vi "Interpolation Example.vi"() -> ()   [LabVIEW 2018]
uses:
  <vilib>/Analysis/1siggen.llb/Ramp Pattern by Samples.vi
  <vilib>/gmath/NI_Gmath.lvlib
  <vilib>/Analysis/NI_AALBase.lvlib
panel:
  out "Raw outputs":cluster{"X":dbl[], "Y":dbl[]}
  in  "samples":i32=256
  in  "method":i32(ring)=1 items=["nearest", "linear", "spline", "cubic Hermite", "Lagrange"]
  in  "Y":dbl[](array[slide]) scale=0.0..1.0
  in  "On/Off":bool
  out "Output Values":cluster{"xi used":dbl[], "yi":dbl[]}(graph)
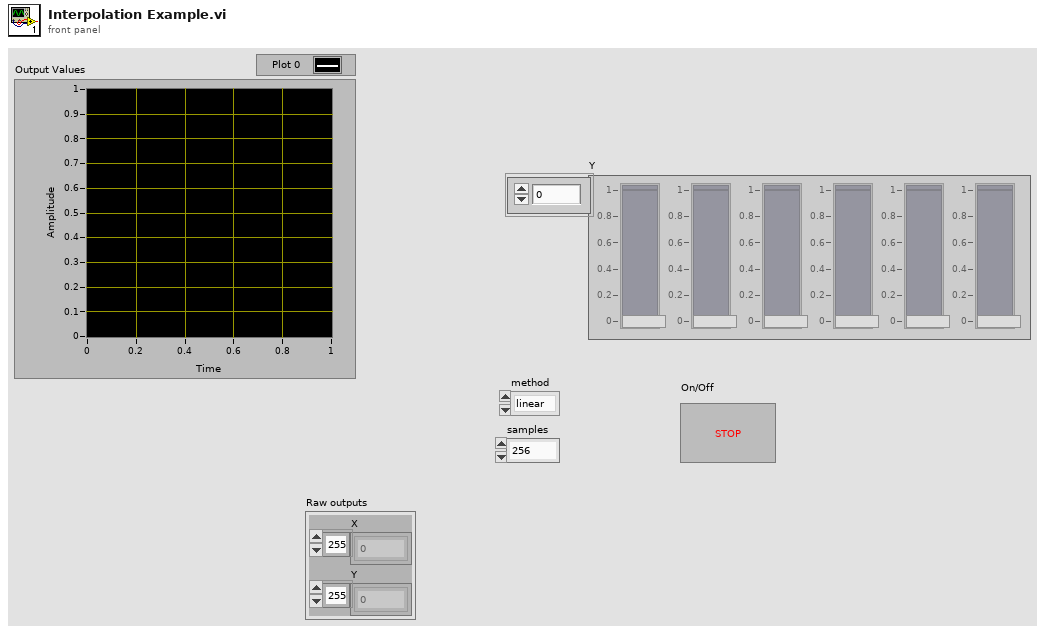
[diagram p1: front panel]
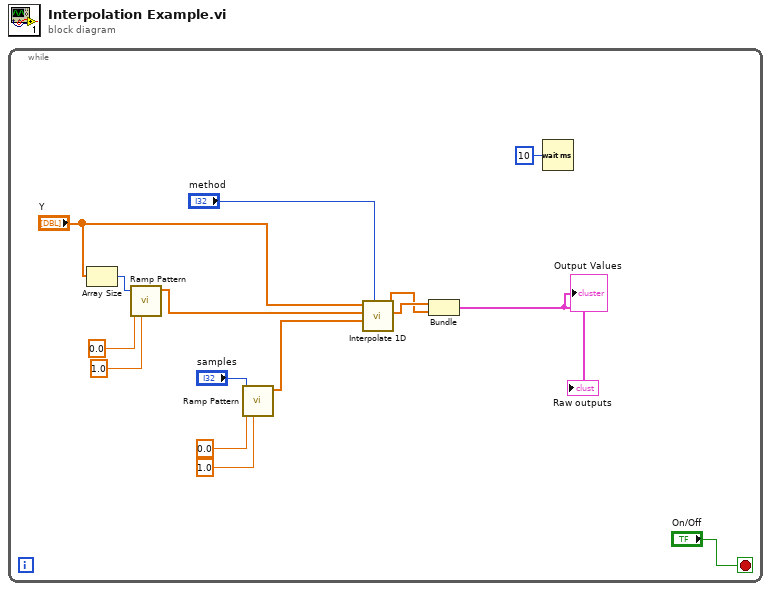
[diagram p0: block diagram]
diagram:
  n1 = while {
    stop <- "On/Off" stop-if-true
    n2 = Array Size(array="Y") -> (size(s)=w1:i32)
    n3 = call-poly <vilib>:"Ramp Pattern.vi"("start"=0.0, "end"=1.0, "samples"=w1) -> ("Ramp Pattern"=w3:dbl[])  [unwired: 7 in, 1 out]
    n4 = call-poly <vilib>:"Ramp Pattern.vi"("start"=0.0, "end"=1.0, "samples"="samples") -> ("Ramp Pattern"=w10:dbl[])  [unwired: 7 in, 1 out]
    n5 = call <vilib>:"Interpolate 1D.vi"("method"="method", "xi"=w10, "X"=w3, "Y"="Y") -> ("xi used"=w14:dbl[], "yi"=w13:dbl[])  [unwired: 5 in, 1 out]
    n6 = Bundle("xi used"=w14, "yi"=w13) -> (→"Output Values" →"Raw outputs":cluster{"xi used":dbl[], "yi":dbl[]})  [unwired: 1 in]
    n7 = Wait (ms)(milliseconds to wait=u32 10) -> ()  [unwired: 1 out]
  }
